vi "LoggingBlock.vi"(7 "Buffer size":i64=1000 min=1 step=1 format="%d data", 8 "error in":errorcluster, 9 "Data In":T2, 11 "Queue Ref":T1) -> (0 "error out":errorcluster)   [LabVIEW 2014]
doc: "<B>Copyright</B>: (c) MHWirth 2015. All rights reserved.\n\nThis subVI, records the shared variable values in a TDMS file. \nIt currently supports the following types of shared variables:\n- Scalars of defined types\n- 1D array of defined types\n- 2D array of defined types\n\n<B>Defined types</B>:\nCode 1. Boolean\nCode 2 to 5. Int8/16/32/64\nCode 6 to 9. UInt8/16/32/64\nCode 10. Double\nCode 11. Single-precision\nCode 12. String"
uses:
  TypeDef/Q1 Message.ctl
  <vilib>/Platform/TimedLoop/XDataNode/timing_clust.ctl
  <vilib>/Platform/TimedLoop/XDataNode/nitl_modes.ctl
  <vilib>/Platform/TimedLoop/XDataNode/wakeup.ctl
  <vilib>/platform/TimedLoop/XDataNode/XDataNode.xnode
  <vilib>/Platform/TimedLoop/XDataNode/XDNodeRunTimeDep.lvlib
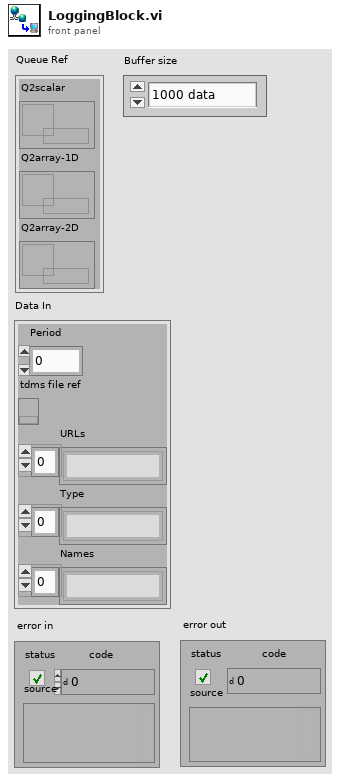
[diagram p1: front panel]
types:
  T1 = cluster{"Q2scalar":refnum<queue>, "Q2array-1D":refnum<queue>, "Q2array-2D":refnum<queue>}
  T2 = cluster{"Period":i64, "tdms file ref":refnum<k34>, "URLs":string[], "Type":string[], "Names":string[]}
  T3 = typedef "Q1 Message.ctl" = cluster{"state":enum16{"initialize 1", "initialize 2", "initialize 3", "initialize 4", "initialize 5", "initialize 6", "initialize 7", "initialize 8", "initialize 9", "Idle", "Preparation 1", "Preparation 2", "Preparation 3", "Preparation 4", "Record", "Stop recording", "Exit", "Defrag", "View", "Create Database", "Update folder setting", "Update Preference", "Update TDMS properties", "CSV Delimiter", "DB Type", "Hidden Processes", "Replace Database", "Logged File Viewer", "Defrag Prompt File", "View Prompt File", "Save to config file", "Open from config file"}, "data":variant}
  T4 = typedef "XDNodeRunTimeDep.lvlib/timing_clust.ctl" = cluster{"Expected End [f-1]":u64, "Actual End [f-1]":u64, "Finished Late? [f-1]":bool, "Expected End [i-1]":u64, "Actual End [i-1]":u64, "Finished Late? [i-1]":bool, "Expected Start [i]":u64, "Actual Start [i]":u64, "Expected Start [f]":u64, "Actual Start [f]":u64, "Source Name":string, "Structure Name":string, "Period":i64, "Deadline":i64, "Offset":i64, "Start":i64, "Priority":i32, "Timeout":i32, "Mode":T5, "Wakeup Reason":T6, "Error":errorcluster, "Source Type":string, "Secondary Source Type":string, "Global End Time":u64, "Global Start Time":u64, "Frame Duration":u64, "Iteration Duration":u64, "Assigned CPU":i32, "I/O Scan Engine Mode":u32}
  T5 = typedef "XDNodeRunTimeDep.lvlib/nitl_modes.ctl" = enum32{"No Change", "Process missed periods, maintain original phase", "Discard missed periods, maintain original phase", "Process missed periods, ignore original phase", "Discard missed periods, ignore original phase"}
  T6 = typedef "XDNodeRunTimeDep.lvlib/wakeup.ctl" = enum32{"Normal", "Aborted", "Asynchronous wakeup", "Timing source error", "Timed loop error", "Timeout"}
  T7 = enum16{"initialize 1", "initialize 2", "initialize 3", "initialize 4", "initialize 5", "initialize 6", "initialize 7", "initialize 8", "initialize 9", "Idle", "Preparation 1", "Preparation 2", "Preparation 3", "Preparation 4", "Record", "Stop recording", "Exit", "Defrag", "View", "Create Database", "Update folder setting", "Update Preference", "Update TDMS properties", "CSV Delimiter", "DB Type", "Hidden Processes", "Replace Database", "Logged File Viewer", "Defrag Prompt File", "View Prompt File", "Save to config file", "Open from config file"}
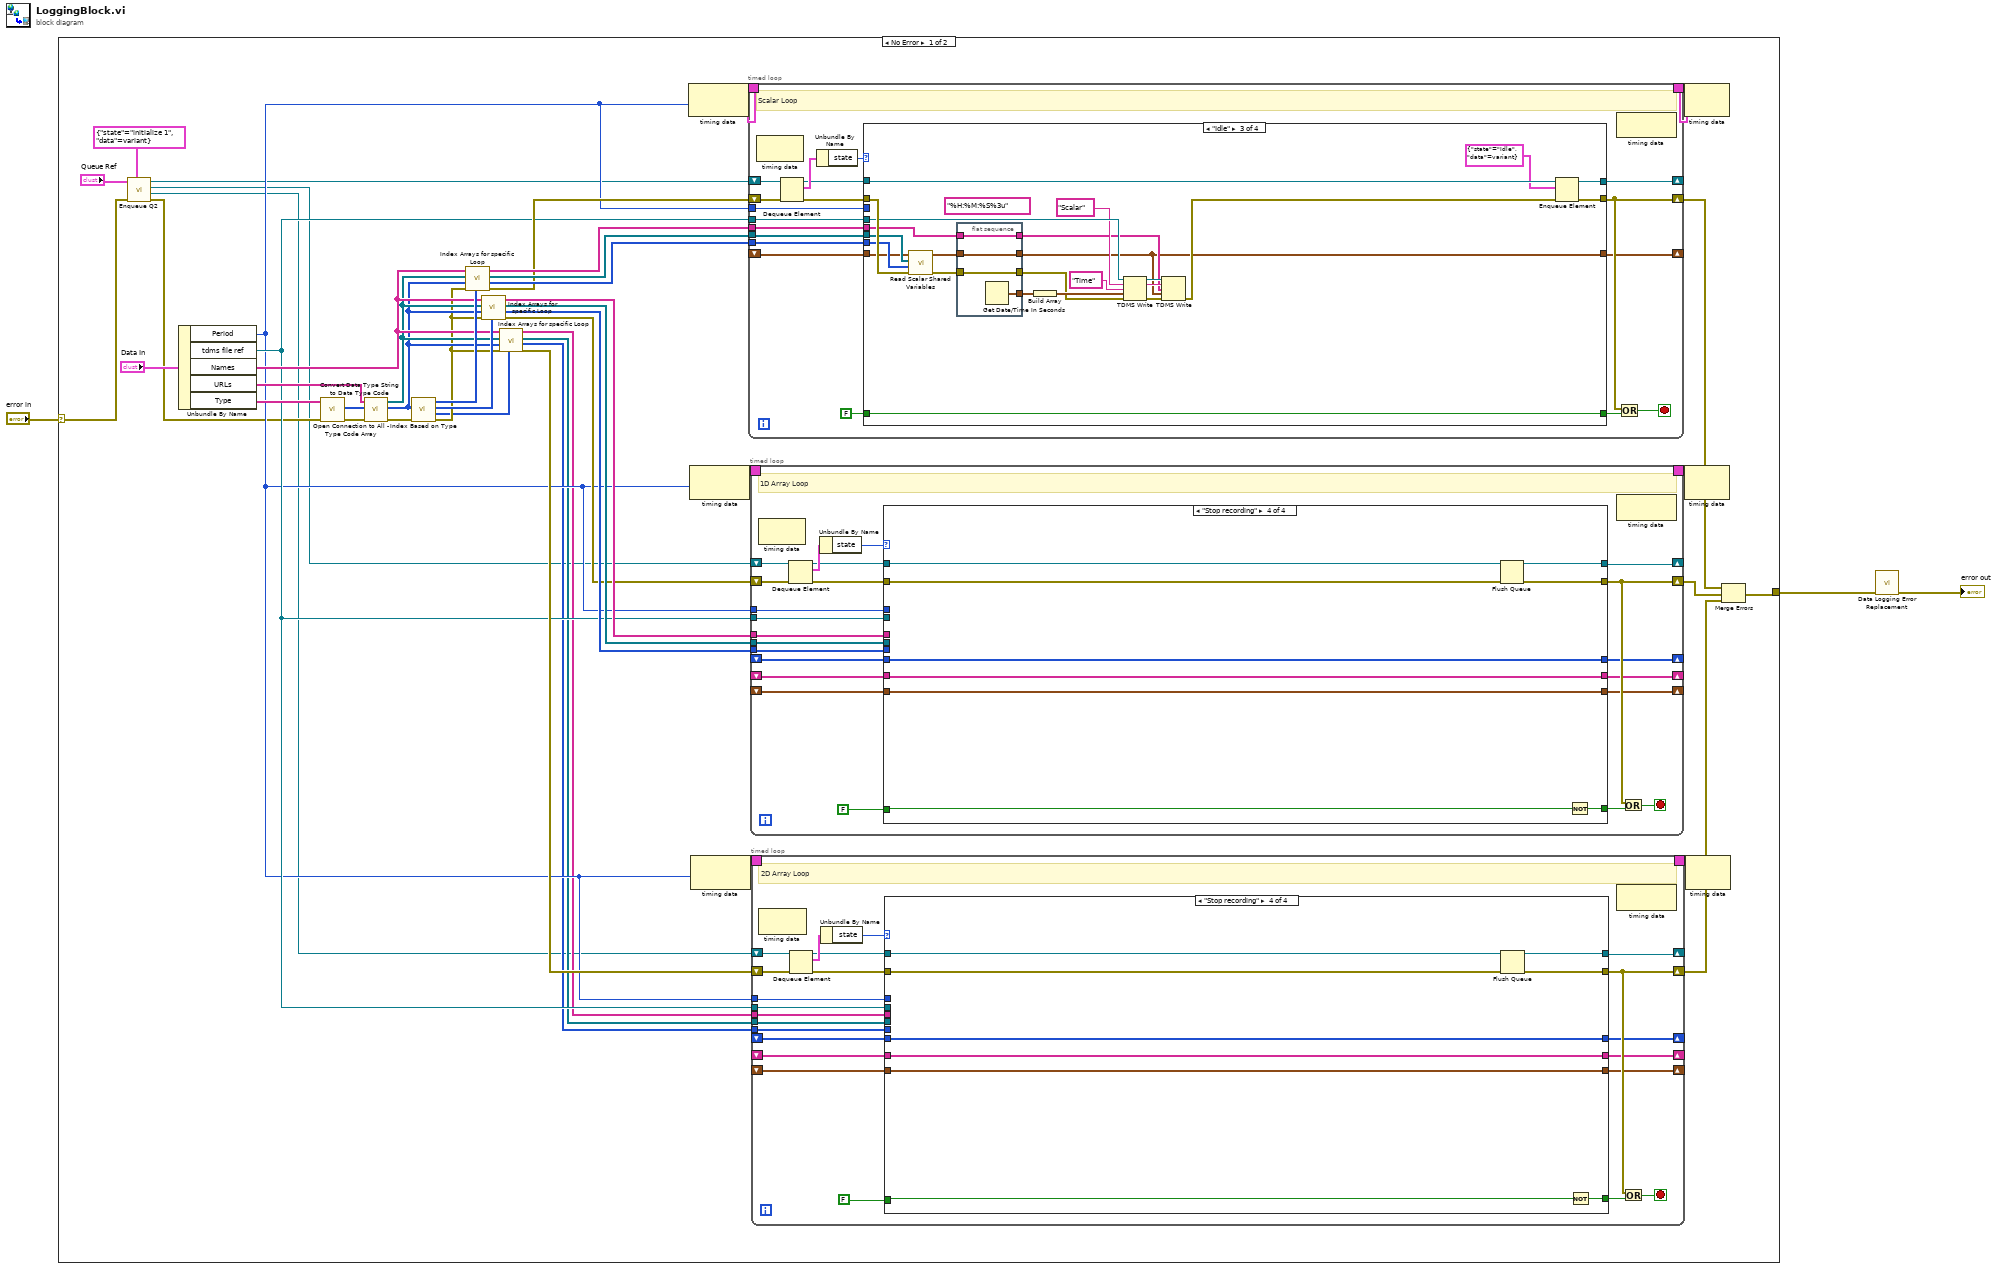
[diagram p0: block diagram]
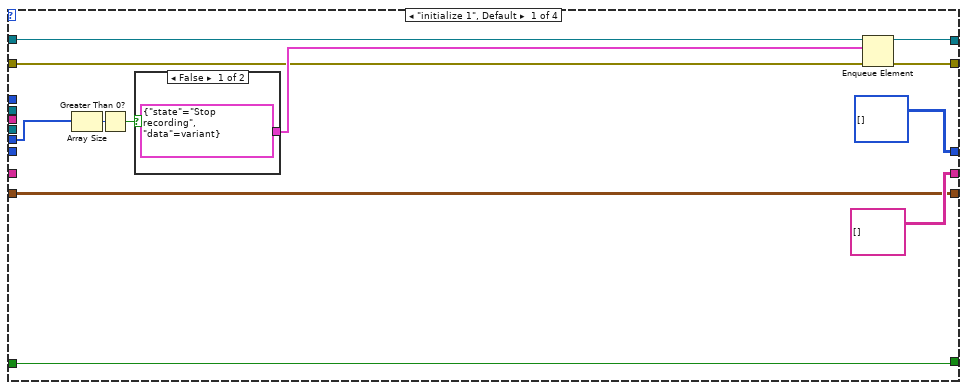
[diagram p2: hidden frame]
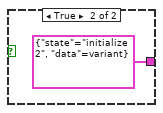
[diagram p3: hidden frame]
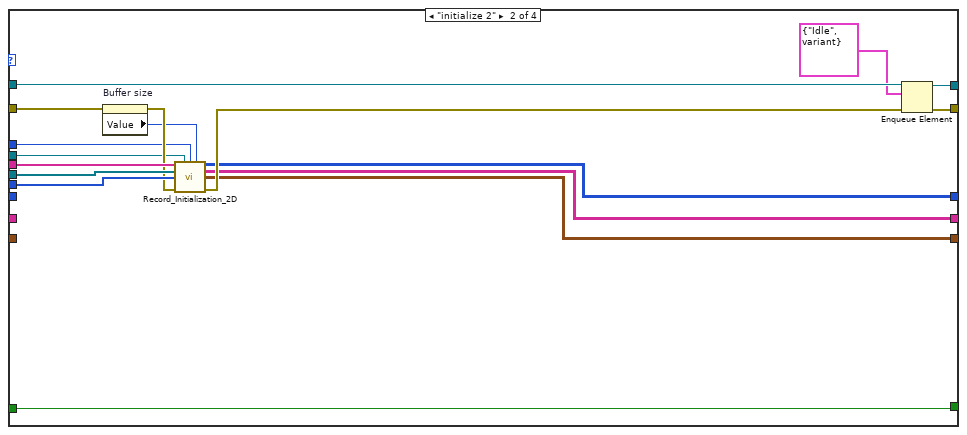
[diagram p4: hidden frame]
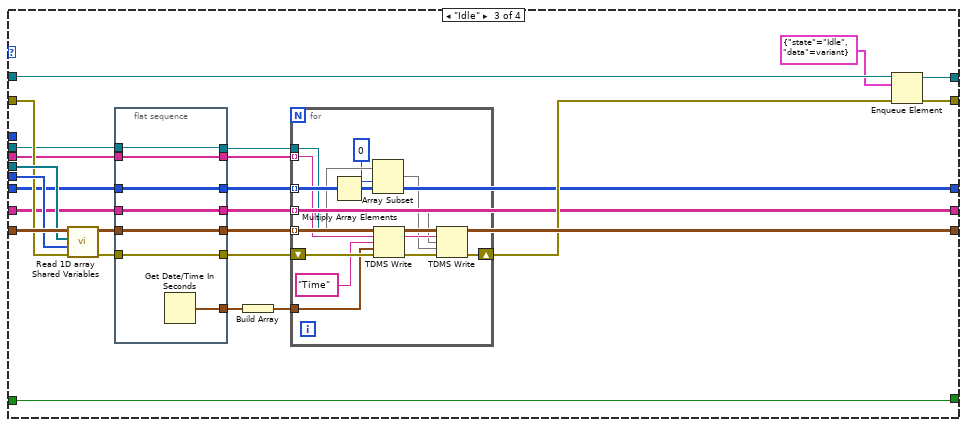
[diagram p5: hidden frame]
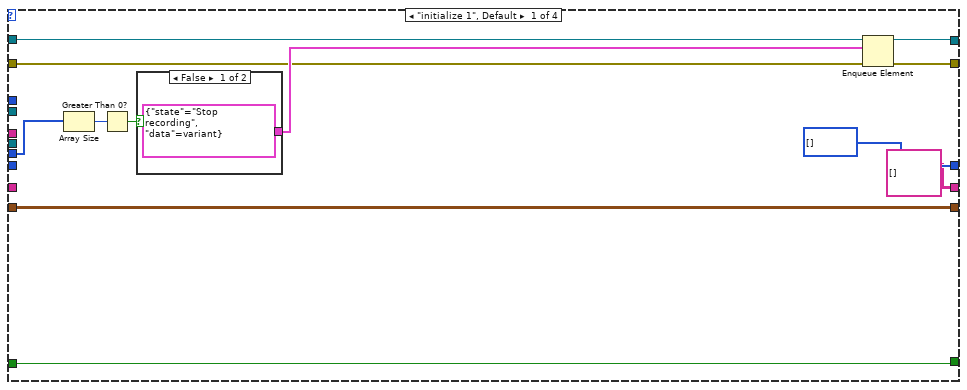
[diagram p6: hidden frame]
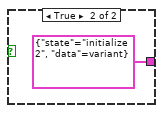
[diagram p7: hidden frame]
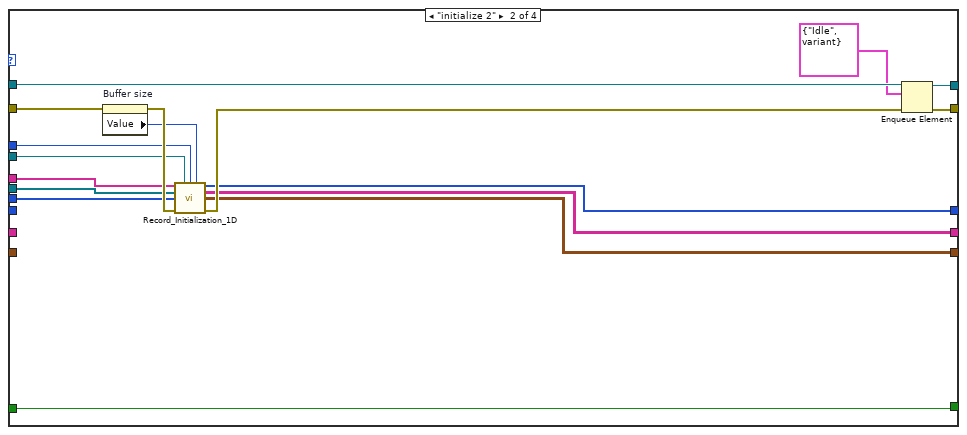
[diagram p8: hidden frame]
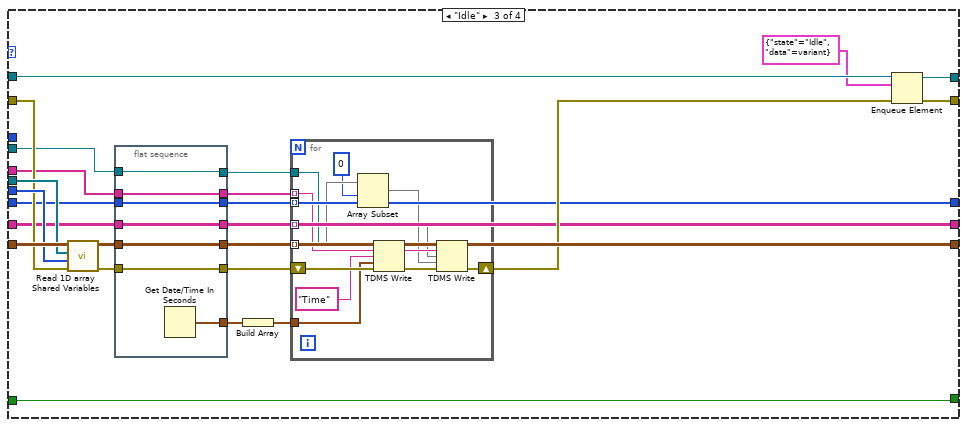
[diagram p9: hidden frame]
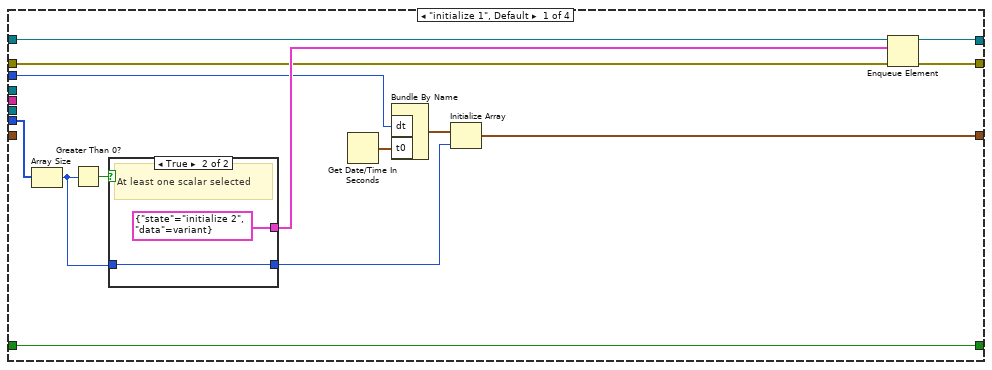
[diagram p10: hidden frame]
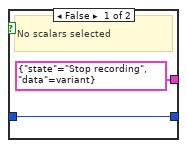
[diagram p11: hidden frame]
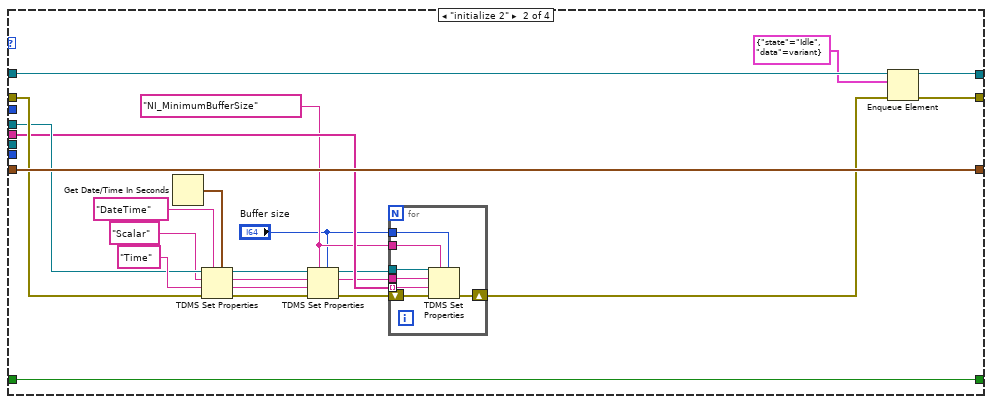
[diagram p12: hidden frame]
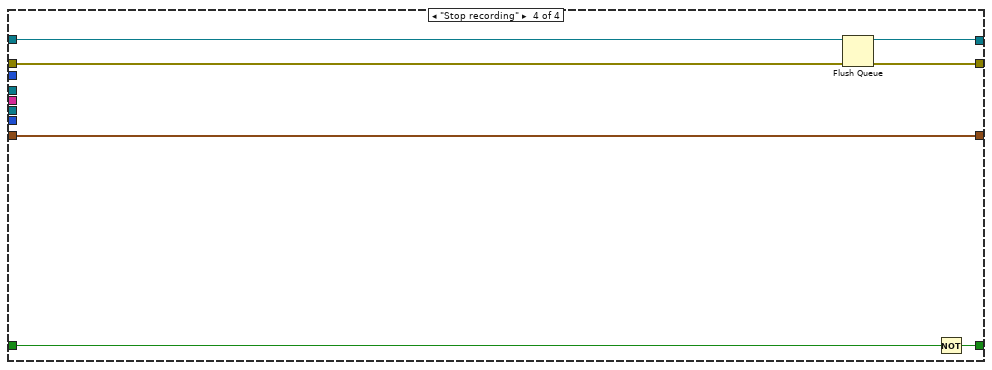
[diagram p13: hidden frame]
diagram:
  n1 = case shown="No Error" "error in" {
    selector: "error in" -> [w9 w382]
    tunnel: [w40 w382] -> w2
    frame No Error {
      n2 = call "Enqueue Q2.vi"("Q1 Message"=T3 {"state"=enum."initialize 1", "data"=variant}, "error in (no error)"=w9, "Queue Ref"="Queue Ref") -> ("error out"=w8:errorcluster, "Q2array-2D"=w5:refnum<queue>, "Q2array-1D"=w6:refnum<queue>, "Q2scalar"=w7:refnum<queue>)  [unwired: 5 in]
      n3 = Unbundle By Name("Data In") -> ("Period"=w14:i64, "tdms file ref"=w15:refnum<k34>, "Names"=w21:string[], "URLs"=w36:string[], "Type"=w37:string[])
      n4 = call "Convert Data Type String to Data Type Code.vi"("Error In"=w8, "Type Array"=w37) -> ("Error Out"=w39:errorcluster, "Type code Array"=w35:i32[])  [unwired: 7 in, 1 out]
      n5 = call "Open Connection to All - Type Code Array.vi"("Error In"=w39, "Type code Array"=w35, "URL array"=w36) -> ("Error Out"=w38:errorcluster, "Type code Array"=w19:i32[], "Array of SV Refnums"=w20:refnum<k21>[])  [unwired: 5 in, 1 out]
      n6 = call "Index Based on Type.vi"("Error In"=w38, "Type code Array"=w19) -> ("Error Out"=w18:errorcluster, "2D array Index"=w17:u32[], "1D array Index"=w25:u32[], "Scalar Index"=w34:u32[])  [unwired: 5 in, 1 out]
      n7 = call "Index Arrays for specific Loop.vi"("Array of Indeces"=w34, "error in (no error)"=w18, "Type code Array"=w19, "Array of SV Refnums"=w20, "Names"=w21) -> ("error out"=w27:errorcluster, "Indexed Type Code"=w31:i32[], "Indexed SV Refnums"=w32:refnum<k21>[], "Indexed Names"=w33:string[])  [unwired: 3 in]
      n8 = call "Index Arrays for specific Loop.vi"("Array of Indeces"=w25, "error in (no error)"=w18, "Type code Array"=w19, "Array of SV Refnums"=w20, "Names"=w21) -> ("error out"=w26:errorcluster, "Indexed Type Code"=w28:i32[], "Indexed SV Refnums"=w29:refnum<k21>[], "Indexed Names"=w30:string[])  [unwired: 3 in]
      n9 = call "Index Arrays for specific Loop.vi"("Array of Indeces"=w17, "error in (no error)"=w18, "Type code Array"=w19, "Array of SV Refnums"=w20, "Names"=w21) -> ("error out"=w16:errorcluster, "Indexed Type Code"=w11:i32[], "Indexed SV Refnums"=w12:refnum<k21>[], "Indexed Names"=w13:string[])  [unwired: 3 in]
      n10 = node-c288(w14) -> (w46:T4)
      n11 = node-c288(w14) -> (w44:T4)
      n12 = node-c288(w14) -> (w24:T4)
      n13 = timed-loop {
        timing: w46 -> [_]
        timing-out: [_] -> w45
        shift-right: [w281] -> w42
        shift-left: w27 -> [w285]
        tunnel: w14 -> [w286]
        shift-right: [w288] -> _
        shift-left: w7 -> [w291]
        shift-right: [w279] -> _
        shift-left: _ -> [w278]
        tunnel: w31 -> [w277]
        tunnel: w32 -> [w275]
        tunnel: w33 -> [w276]
        tunnel: w15 -> [w287]
        stop <- w280 stop-if-true
        # "Scalar Loop"
        n14 = node-c288() -> ()  [unwired: 1 in, 1 out]
        n15 = Dequeue Element(queue=w291, error in (no error)=w285) -> (queue out=w289:refnum<queue>, element=w292:T3, error out=w284:errorcluster)  [unwired: 1 in, 1 out]
        n16 = Unbundle By Name(w292) -> ("state"=w290:T7)
        n17 = case shown="\"Idle\"" w290 {
          tunnel: w284 -> [w294 w320 w354 w374]
          tunnel: [w302 w331 w358 w373] -> w281
          tunnel: w289 -> [w306 w333 w362 w375]
          tunnel: [w305 w332 w361 w372] -> w288
          tunnel: [w301 w330 w355 w371] -> w282
          tunnel: w287 -> [_ w319 w348 _]
          tunnel: w286 -> [w298 _ _ _]
          tunnel: FALSE -> [w301 w330 w355 w370]
          tunnel: [w300 w325 w342 w369] -> w279
          tunnel: w278 -> [_ w325 w341 w369]
          tunnel: w277 -> [w293 _ w352 _]
          tunnel: w276 -> [_ w316 w344 _]
          tunnel: w275 -> [_ _ w353 _]
          frame "initialize 1", Default {
            n18 = Array Size(array=w293) -> (size(s)=w296:i32)
            n19 = Greater Than 0?(x=w296) -> (x > 0?=w304:bool)
            n20 = case shown="True" w304 {
              tunnel: [T3 {"state"=enum."Stop recording", "data"=variant} ("Q1 Message") T3 {"state"=enum."initialize 2", "data"=variant} ("Q1 Message")] -> w303
              tunnel: w296 -> [w307 w309]
              tunnel: [w307 w309] -> w295
              frame False {
                # "No scalars selected"
              }
              frame True {
                # "At least one scalar selected"
              }
            }
            n21 = Get Date/Time In Seconds() -> (seconds since 1Jan1904=w297:timestamp)
            n22 = Bundle By Name("dt"=w298, "t0"=w297) -> (w299:waveform(dbl))  [unwired: 1 in]
            n23 = Initialize Array(w299, w295) -> (w300:waveform(dbl)[])
            n24 = Enqueue Element(queue=w306, element=w303, error in (no error)=w294) -> (queue out=w305:refnum<queue>, error out=w302:errorcluster)  [unwired: 1 in, 1 out]
          }
          frame "initialize 2" {
            w313 = "NI_MinimumBufferSize"
            n25 = Get Date/Time In Seconds() -> (seconds since 1Jan1904=w328:timestamp)
            n26 = TDMS Set Properties(5:w328, 7:"DateTime" ("property names"), 8:w320, 9:"Time", 10:"Scalar", 11:w319) -> (0:w321:errorcluster, 1:w322:string, 2:w323:string, 3:w324:refnum<k34>)
            n27 = TDMS Set Properties(5:"Buffer size", 7:w313, 8:w321, 9:w322, 10:w323, 11:w324) -> (0:w317:errorcluster, 2:w315:string, 3:w314:refnum<k34>)  [unwired: 1 out]
            n28 = for {
              shift-right: [w339] -> w311
              shift-left: w317 -> [w340]
              tunnel: w316 -> [w338] mode=indexing
              tunnel: w315 -> [w337]
              tunnel: w314 -> [w336]
              tunnel: w313 -> [w335]
              tunnel: "Buffer size" -> [w334]
              n29 = TDMS Set Properties(5:w334, 7:w335, 8:w340, 9:w338, 10:w337, 11:w336) -> (0:w339:errorcluster)  [unwired: 3 out]
            }
            n30 = Enqueue Element(queue=w333, element=T3 {"state"=enum."Idle", "data"=variant} ("Q1 Message"), error in (no error)=w311) -> (queue out=w332:refnum<queue>, error out=w331:errorcluster)  [unwired: 1 in, 1 out]
          }
          frame "Idle" {
            (unwired) "%H:%M:%S%3u" ("time format string (%c)")
            n31 = call "Read Scalar Shared Variables.vi"("Error In"=w354, "Array of Type code"=w352, "Array of SV Refnums"=w353, "Waveform Array in"=w341) -> ("Error Out"=w351:errorcluster, "Waveform Array out"=w350:waveform(dbl)[])  [unwired: 6 in]
            n32 = flat-sequence {
              tunnel: [w368] -> w357
              tunnel: w351 -> [w367]
              tunnel: [w367] -> w349
              tunnel: w350 -> [w366]
              tunnel: [w366] -> w342
              tunnel: w344 -> [w365]
              tunnel: [w365] -> w343
              frame #0 {
                n33 = Get Date/Time In Seconds() -> (seconds since 1Jan1904=w368:timestamp)
              }
            }
            n34 = Build Array(w357) -> (w356:timestamp[])
            n35 = TDMS Write(0:w348, 5:"Scalar", 7:"Time", 9:w356, 11:w349) -> (4:w347:refnum<k34>, 6:w345:string, 15:w363:errorcluster)  [unwired: 1 in, 1 out]
            n36 = TDMS Write(0:w347, 5:w345, 7:w343, 9:w342, 11:w363) -> (15:w359:errorcluster)  [unwired: 1 in, 3 out]
            n37 = Enqueue Element(queue=w362, element=T3 {"state"=enum."Idle", "data"=variant} ("Q1 Message"), error in (no error)=w359) -> (queue out=w361:refnum<queue>, error out=w358:errorcluster)  [unwired: 1 in, 1 out]
          }
          frame "Stop recording" {
            n38 = Flush Queue(queue=w375, error in (no error)=w374) -> (queue out=w372:refnum<queue>, error out=w373:errorcluster)  [unwired: 1 out]
            n39 = Not(x=w370) -> (.not. x?=w371:bool)
          }
        }
        n40 = node-c288() -> ()  [unwired: 1 in, 1 out]
        n41 = Or(x=w281, y=w282) -> (x .or. y?=w280:bool)
      }
      n42 = timed-loop {
        timing: w44 -> [_]
        timing-out: [_] -> w43
        shift-right: [w172] -> w41
        shift-left: w26 -> [w175]
        tunnel: w14 -> [w177]
        shift-right: [w179] -> _
        shift-left: w6 -> [w182]
        tunnel: w15 -> [w178]
        tunnel: w28 -> [w168]
        tunnel: w30 -> [w169]
        tunnel: w29 -> [w170]
        shift-right: [w167] -> _
        shift-left: _ -> [w166]
        shift-right: [w165] -> _
        shift-left: _ -> [w164]
        shift-right: [w163] -> _
        shift-left: _ -> [w162]
        stop <- w171 stop-if-true
        # "1D Array Loop"
        n43 = node-c288() -> ()  [unwired: 1 in, 1 out]
        n44 = Dequeue Element(queue=w182, error in (no error)=w175) -> (queue out=w180:refnum<queue>, element=w183:T3, error out=w176:errorcluster)  [unwired: 1 in, 1 out]
        n45 = Unbundle By Name(w183) -> ("state"=w181:T7)
        n46 = case shown="\"Stop recording\"" w181 {
          tunnel: w176 -> [w188 w213 w230 w267]
          tunnel: w178 -> [_ w204 w224 _]
          tunnel: [w191 w211 w235 w266] -> w172
          tunnel: w180 -> [w195 w212 w238 w268]
          tunnel: [w194 w210 w237 w265] -> w179
          tunnel: w177 -> [_ w203 _ _]
          tunnel: FALSE -> [w190 w208 w234 w264]
          tunnel: [w190 w208 w234 w263] -> w173
          tunnel: w170 -> [_ w206 w232 _]
          tunnel: w169 -> [_ w207 w225 _]
          tunnel: w168 -> [w189 w205 w231 _]
          tunnel: [w184 w198 w219 w260] -> w167
          tunnel: w166 -> [w184 _ w233 w260]
          tunnel: [string[][] [] w199 w217 w261] -> w165
          tunnel: w164 -> [_ _ w226 w261]
          tunnel: [i32[] [] w200 w215 w262] -> w163
          tunnel: w162 -> [_ _ w216 w262]
          frame "initialize 1", Default {
            n47 = Array Size(array=w189) -> (size(s)=w187:i32)
            n48 = Greater Than 0?(x=w187) -> (x > 0?=w193:bool)
            n49 = case shown="False" w193 {
              tunnel: [T3 {"state"=enum."Stop recording", "data"=variant} ("Q1 Message") T3 {"state"=enum."initialize 2", "data"=variant} ("Q1 Message")] -> w192
              frame False {
              }
              frame True {
              }
            }
            n50 = Enqueue Element(queue=w195, element=w192, error in (no error)=w188) -> (queue out=w194:refnum<queue>, error out=w191:errorcluster)  [unwired: 1 in, 1 out]
          }
          frame "initialize 2" {
            n51 = property on="Buffer size" class="DigNum (strict)"(error in=w213) -> (error out=w214:errorcluster, "Value"=w202:i64)  [unwired: 1 in, 1 out]
            n52 = call "Record_Initialization_1D.vi"("Indexed Names"=w207, "Refnum in"=w204, "Period"=w203, "Buffer size"=w202, "Indexed SV Refnums"=w206, "Indexed Type Code"=w205, "error in (no error)"=w214) -> ("Array of sizes"=w200:i32[], "Array of channel names"=w199:string[][], "Array of 1D waveforms"=w198:waveform(dbl)[][], "error out"=w201:errorcluster)  [unwired: 5 in]
            n53 = Enqueue Element(queue=w212, element=T3 {"state"=enum."Idle", "data"=variant} ("Q1 Message"), error in (no error)=w201) -> (queue out=w210:refnum<queue>, error out=w211:errorcluster)  [unwired: 1 in, 1 out]
          }
          frame "Idle" {
            n54 = call "Read 1D array Shared Variables.vi"("Error In"=w230, "Array of Type code"=w231, "Array of SV Refnums"=w232, "Waveform Array in"=w233) -> ("Error Out"=w228:errorcluster, "Waveform Array out"=w229:waveform(dbl)[][])  [unwired: 6 in]
            n55 = flat-sequence {
              tunnel: [w259] -> w219
              tunnel: w229 -> [w259]
              tunnel: w228 -> [w258]
              tunnel: [w258] -> w220
              tunnel: [w257] -> w227
              tunnel: [w256] -> w217
              tunnel: w226 -> [w256]
              tunnel: [w255] -> w223
              tunnel: w225 -> [w255]
              tunnel: [w254] -> w222
              tunnel: w224 -> [w254]
              tunnel: [w253] -> w215
              tunnel: w216 -> [w253]
              frame #0 {
                n56 = Get Date/Time In Seconds() -> (seconds since 1Jan1904=w257:timestamp)
              }
            }
            n57 = Build Array(w227) -> (w221:timestamp[])
            n58 = for {
              tunnel: w217 -> [w244] mode=indexing
              tunnel: w219 -> [w242] mode=indexing
              tunnel: w223 -> [w251] mode=indexing
              tunnel: w222 -> [w250]
              tunnel: w221 -> [w245]
              shift-right: [w243] -> w218
              shift-left: w220 -> [w252]
              tunnel: w215 -> [w241] mode=indexing
              n59 = Array Subset(array=w242, index=0, length=w241) -> (w239:waveform(dbl)[])
              n60 = TDMS Write(0:w250, 5:w251, 7:"Time", 9:w245, 11:w252) -> (4:w249:refnum<k34>, 6:w248:string, 15:w247:errorcluster)  [unwired: 1 in, 1 out]
              n61 = TDMS Write(0:w249, 5:w248, 7:w244, 9:w239, 11:w247) -> (15:w243:errorcluster)  [unwired: 1 in, 3 out]
            }
            n62 = Enqueue Element(queue=w238, element=T3 {"state"=enum."Idle", "data"=variant} ("Q1 Message"), error in (no error)=w218) -> (queue out=w237:refnum<queue>, error out=w235:errorcluster)  [unwired: 1 in, 1 out]
          }
          frame "Stop recording" {
            n63 = Flush Queue(queue=w268, error in (no error)=w267) -> (queue out=w265:refnum<queue>, error out=w266:errorcluster)  [unwired: 1 out]
            n64 = Not(x=w264) -> (.not. x?=w263:bool)
          }
        }
        n65 = node-c288() -> ()  [unwired: 1 in, 1 out]
        n66 = Or(x=w172, y=w173) -> (x .or. y?=w171:bool)
      }
      n67 = timed-loop {
        timing: w24 -> [_]
        timing-out: [_] -> w23
        shift-right: [w58] -> w22
        shift-left: w16 -> [w61]
        tunnel: w14 -> [w63]
        shift-right: [w65] -> _
        shift-left: w5 -> [w68]
        tunnel: w15 -> [w64]
        tunnel: w11 -> [w54]
        tunnel: w13 -> [w55]
        tunnel: w12 -> [w56]
        shift-right: [w53] -> _
        shift-left: _ -> [w52]
        shift-right: [w51] -> _
        shift-left: _ -> [w50]
        shift-right: [w49] -> _
        shift-left: _ -> [w48]
        stop <- w57 stop-if-true
        # "2D Array Loop"
        n68 = node-c288() -> ()  [unwired: 1 in, 1 out]
        n69 = Dequeue Element(queue=w68, error in (no error)=w61) -> (queue out=w66:refnum<queue>, element=w69:T3, error out=w62:errorcluster)  [unwired: 1 in, 1 out]
        n70 = Unbundle By Name(w69) -> ("state"=w67:T7)
        n71 = case shown="\"Stop recording\"" w67 {
          tunnel: w62 -> [w74 w100 w116 w154]
          tunnel: w64 -> [_ w90 w110 _]
          tunnel: [w77 w98 w121 w153] -> w58
          tunnel: w66 -> [w81 w99 w124 w155]
          tunnel: [w80 w97 w123 w152] -> w65
          tunnel: w63 -> [_ w84 _ _]
          tunnel: FALSE -> [w76 w95 w120 w151]
          tunnel: [w76 w95 w120 w150] -> w59
          tunnel: w56 -> [_ w93 w118 _]
          tunnel: w55 -> [_ w94 w111 _]
          tunnel: w54 -> [w75 w92 w117 _]
          tunnel: [w70 w85 w105 w147] -> w53
          tunnel: w52 -> [w70 _ w119 w147]
          tunnel: [string[][] [] w86 w103 w148] -> w51
          tunnel: w50 -> [_ _ w112 w148]
          tunnel: [i32[][] [] w87 w101 w149] -> w49
          tunnel: w48 -> [_ _ w102 w149]
          frame "initialize 1", Default {
            n72 = Array Size(array=w75) -> (size(s)=w73:i32)
            n73 = Greater Than 0?(x=w73) -> (x > 0?=w79:bool)
            n74 = case shown="False" w79 {
              tunnel: [T3 {"state"=enum."Stop recording", "data"=variant} ("Q1 Message") T3 {"state"=enum."initialize 2", "data"=variant} ("Q1 Message")] -> w78
              frame False {
              }
              frame True {
              }
            }
            n75 = Enqueue Element(queue=w81, element=w78, error in (no error)=w74) -> (queue out=w80:refnum<queue>, error out=w77:errorcluster)  [unwired: 1 in, 1 out]
          }
          frame "initialize 2" {
            n76 = property on="Buffer size" class="DigNum (strict)"(error in=w100) -> (error out=w91:errorcluster, "Value"=w89:i64)  [unwired: 1 in, 1 out]
            n77 = call "Record_Initialization_2D.vi"("Indexed Names"=w94, "Refnum in"=w90, "Period"=w84, "Buffer size"=w89, "Indexed SV Refnums"=w93, "Indexed Type Code"=w92, "error in (no error)"=w91) -> ("2D Array of sizes"=w87:i32[][], "Array of channel names"=w86:string[][], "Array of 1D waveforms"=w85:waveform(dbl)[][], "error out"=w88:errorcluster)  [unwired: 5 in]
            n78 = Enqueue Element(queue=w99, element=T3 {"state"=enum."Idle", "data"=variant} ("Q1 Message"), error in (no error)=w88) -> (queue out=w97:refnum<queue>, error out=w98:errorcluster)  [unwired: 1 in, 1 out]
          }
          frame "Idle" {
            n79 = call "Read 1D array Shared Variables.vi"("Error In"=w116, "Array of Type code"=w117, "Array of SV Refnums"=w118, "Waveform Array in"=w119) -> ("Error Out"=w114:errorcluster, "Waveform Array out"=w115:waveform(dbl)[][])  [unwired: 6 in]
            n80 = flat-sequence {
              tunnel: [w146] -> w105
              tunnel: w115 -> [w146]
              tunnel: w114 -> [w145]
              tunnel: [w145] -> w106
              tunnel: [w144] -> w113
              tunnel: [w143] -> w103
              tunnel: w112 -> [w143]
              tunnel: [w142] -> w109
              tunnel: w111 -> [w142]
              tunnel: [w141] -> w108
              tunnel: w110 -> [w141]
              tunnel: [w140] -> w101
              tunnel: w102 -> [w140]
              frame #0 {
                n81 = Get Date/Time In Seconds() -> (seconds since 1Jan1904=w144:timestamp)
              }
            }
            n82 = Build Array(w113) -> (w107:timestamp[])
            n83 = for {
              tunnel: w103 -> [w131] mode=indexing
              tunnel: w105 -> [w129] mode=indexing
              tunnel: w109 -> [w138] mode=indexing
              tunnel: w108 -> [w137]
              tunnel: w107 -> [w132]
              shift-right: [w130] -> w104
              shift-left: w106 -> [w139]
              tunnel: w101 -> [w125] mode=indexing
              n84 = Multiply Array Elements(1:w125) -> (0:w126:i32)
              n85 = Array Subset(array=w129, index=0, length=w126) -> (w127:waveform(dbl)[])
              n86 = TDMS Write(0:w137, 5:w138, 7:"Time", 9:w132, 11:w139) -> (4:w136:refnum<k34>, 6:w135:string, 15:w134:errorcluster)  [unwired: 1 in, 1 out]
              n87 = TDMS Write(0:w136, 5:w135, 7:w131, 9:w127, 11:w134) -> (15:w130:errorcluster)  [unwired: 1 in, 3 out]
            }
            n88 = Enqueue Element(queue=w124, element=T3 {"state"=enum."Idle", "data"=variant} ("Q1 Message"), error in (no error)=w104) -> (queue out=w123:refnum<queue>, error out=w121:errorcluster)  [unwired: 1 in, 1 out]
          }
          frame "Stop recording" {
            n89 = Flush Queue(queue=w155, error in (no error)=w154) -> (queue out=w152:refnum<queue>, error out=w153:errorcluster)  [unwired: 1 out]
            n90 = Not(x=w151) -> (.not. x?=w150:bool)
          }
        }
        n91 = node-c288() -> ()  [unwired: 1 in, 1 out]
        n92 = Or(x=w58, y=w59) -> (x .or. y?=w57:bool)
      }
      n93 = node-c288(w45) -> ()  [unwired: 1 out]
      n94 = node-c288(w43) -> ()  [unwired: 1 out]
      n95 = node-c288(w23) -> ()  [unwired: 1 out]
      n96 = Merge Errors(w42, w41, w22) -> (w40:errorcluster)
    }
    frame Error {
    }
  }
  n97 = call "Data Logging Error Replacement.vi"("error in (no error)"=w2) -> ("error out"=→"error out":errorcluster)  [unwired: 10 in]
